vi "Get Multi Instrument Handler.vi"(8 "error in (no error)":errorcluster, 10 "Msg":refnum<class "Multi Instrument Msg.lvclass">, 11 "Instrument Handler in":refnum<class "Instrument Handler.lvclass">) -> (0 "error out":errorcluster, 1 "Success?":bool, 2 "Enqueuer":refnum<class "Message Enqueuer.lvclass">, 3 "Instrument Handler out":refnum<class "Instrument Handler.lvclass">)   [LabVIEW 2020, in "Instrument Handler.lvlib" / "Instrument Handler.lvclass"]
doc: "Get the enqueuer of a Multi Instrument Handler from the Instrument Handler. New Multi INstrument Handlers will be launched when needed.\nHandlers are first found by Msg base name and and then any idle Handler. If none are idle a new is launched."
uses:
  Instrument Handler.lvclass
  Messages/Multi Instrument Msg/Multi Instrument Msg.lvclass
  PPL/HDH.Actor Framework.Core.Actor.lvlibp/1abvi3w/vi.lib/ActorFramework/Message Enqueuer/Message Enqueuer.lvclass
  Instrument Handler.lvclass/Instrument Handler.ctl
  Multi Instrument Handler/Multi Instrument Handler.lvclass/Multi Instrument Handler.ctl
  Controls/Ctl_MultiInstruments.ctl
  Multi Instrument Handler/Multi Instrument Handler.lvclass
  PPL/HDH.Data.Generic.lvlibp
  PPL/HDH.Actor Framework.Core.Actor.lvlibp/1abvi3w/vi.lib/ActorFramework/Actor/Actor.lvclass
  Instrument Handler.lvlib
  C:/Current projects/WS/PPL/HDH.Actor Framework.Core.Actor.lvlibp/1abvi3w/vi.lib/ActorFramework/Actor/Actor.lvclass
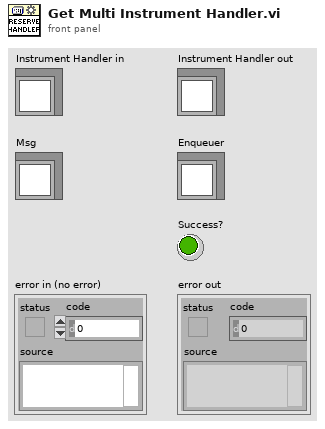
[diagram p1: front panel]
types:
  T1 = typedef "Instrument Handler.lvlib/Ctl_MultiInstruments.ctl" = cluster{"Callers":i32, "Msg Name":string, "Enqueuer":refnum<class "Message Enqueuer.lvclass">}
  T2 = typedef "Semaphore RefNum" = refnum<k1>
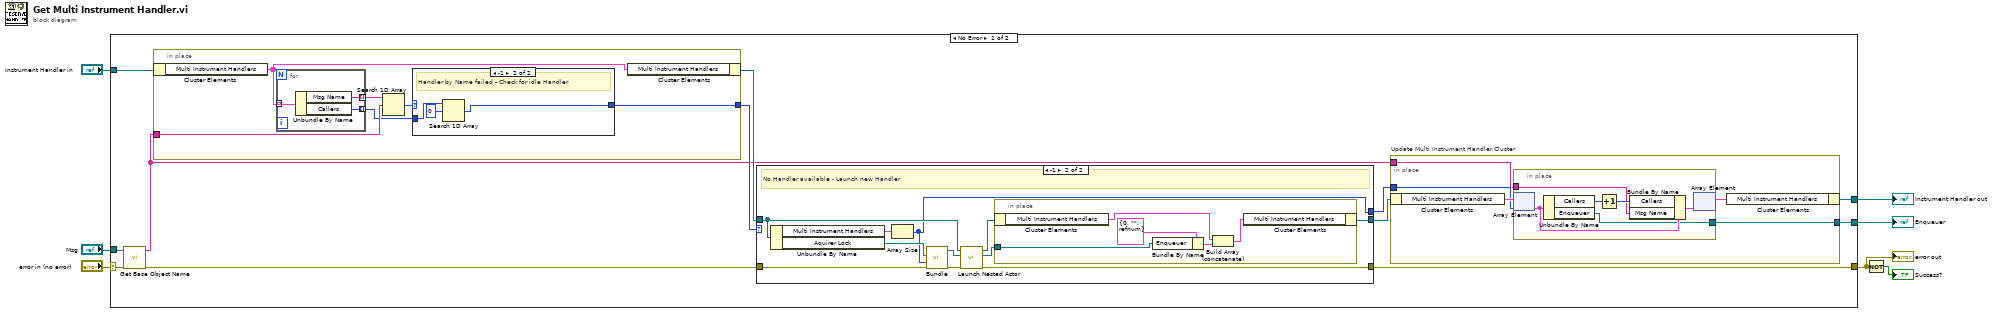
[diagram p0: block diagram]
diagram:
  n1 = case shown="No Error" "error in (no error)" {
    selector: "error in (no error)" -> [w17 w64]
    tunnel: [w14 w64] -> w2
    tunnel: [w11 w63] -> w5
    tunnel: "Instrument Handler in" -> [w19 w63]
    tunnel: "Msg" -> [w18 _]
    tunnel: [w8 _] -> w3
    frame No Error {
      n2 = call "Get Base Object Name.vi"("error in (no error)"=w17, "Object in"=w18) -> ("error out"=w13:errorcluster, "Base class name"=w9:string)  [unwired: 8 in]
      n3 = in-place {
        in-place-border: w9 -> [w54]
        in-place-border: [w50] -> w16
        n4 = in-place-cluster #1(w19) -> ("Multi Instrument Handlers"=w51:T1[])
        n5 = for {
          tunnel: w51 -> [w62] mode=indexing
          tunnel: [w61] -> w55 mode=indexing
          tunnel: [w60] -> w52 mode=indexing
          n6 = Unbundle By Name(w62) -> ("Msg Name"=w61:string, "Callers"=w60:i32)
        }
        n7 = Search 1D Array(1D array=w55, element=w54) -> (index of element=w53:i32)  [unwired: 1 in]
        n8 = case shown="-1" w53 {
          selector: w53 -> [w56 _]
          tunnel: w52 -> [_ w59]
          tunnel: [w56 w57] -> w50
          frame Default {
            # "Handler found by name"
          }
          frame -1 {
            # "Handler by Name failed - Check for idle Handler"
            n9 = Search 1D Array(1D array=w59, element=0) -> (index of element=w57:i32)  [unwired: 1 in]
          }
        }
        n10 = in-place-cluster #1("Multi Instrument Handlers"=w51) -> (w15:refnum<class "Instrument Handler.lvclass">)
      }
      n11 = case shown="-1" w16 {
        selector: w16 -> [w31 _]
        tunnel: [w33 w35] -> w12
        tunnel: w15 -> [w33 w42]
        tunnel: [w32 w34] -> w14
        tunnel: w13 -> [w32 w40]
        tunnel: [w31 w36] -> w10
        frame Default {
          # "Handler found - No action"
        }
        frame -1 {
          # "No Handler available - Launch new Handler"
          n12 = Unbundle By Name(w42) -> ("Multi Instrument Handlers"=w44:T1[], "Aquirer Lock"=w43:T2)
          n13 = Array Size(array=w44) -> (size(s)=w36:i32)
          n14 = call "Bundle.vi"("error in (no error)"=w40, "Hander Index"=w36, "Aquirer Lock"=w43) -> ("error out"=w39:errorcluster, "Multi Instrument Handler out"=w41:refnum<class "Multi Instrument Handler.lvclass">)  [unwired: 7 in]
          n15 = call "Launch Nested Actor.vi"("error in (no error)"=w39, "Nested Actor"=w41, "Caller Actor in"=w42) -> ("error out"=w34:errorcluster, "Nested Actor's Enqueuer"=w37:refnum<class "Message Enqueuer.lvclass">, "Caller Actor out"=w38:refnum<class "Instrument Handler.lvclass">)  [unwired: 6 in]
          n16 = in-place {
            in-place-border: w37 -> [w48]
            n17 = in-place-cluster #2(w38) -> ("Multi Instrument Handlers"=w47:T1[])
            n18 = Bundle By Name(cluster=T1 {"Callers"=0, "Msg Name"="", "Enqueuer"=refnum} ("Instrument cluster"), "Enqueuer"=w48) -> (w46:T1)
            n19 = Build Array (concatenate)(w47, w46) -> (w45:T1[])
            n20 = in-place-cluster #2("Multi Instrument Handlers"=w45) -> (w35:refnum<class "Instrument Handler.lvclass">)
          }
        }
      }
      n21 = in-place "Update Multi Instrument Handler Cluster" {
        in-place-border: w10 -> [w22]
        in-place-border: w9 -> [w21]
        in-place-border: [w20] -> w8
        n22 = in-place-cluster #3(w12) -> ("Multi Instrument Handlers"=w24:T1[])
        n23 = in-place {
          in-place-border: w21 -> [w26]
          in-place-border: [w25] -> w20
          n24 = in-place-array #4(w24, w22) -> (w30:T1)
          n25 = Unbundle By Name(w30) -> ("Callers"=w29:i32, "Enqueuer"=w25:refnum<class "Message Enqueuer.lvclass">)
          n26 = Increment(x=w29) -> (x+1=w28:i32)
          n27 = Bundle By Name(cluster=w30, "Callers"=w28, "Msg Name"=w26) -> (w27:T1)
          n28 = in-place-array #4(w27) -> (w23:T1[])  [unwired: 1 out]
        }
        n29 = in-place-cluster #3("Multi Instrument Handlers"=w23) -> (w11:refnum<class "Instrument Handler.lvclass">)
      }
    }
    frame Error {
    }
  }
  "error out" <- w2
  "Instrument Handler out" <- w5
  "Enqueuer" <- w3
  n30 = Not(x=w2) -> (.not. x?=→"Success?":bool)
